vi "Convert Enum to Image.vi"(6 "picture background":picture, 8 "error in":errorcluster, 11 "Graphics":T1="info") -> (0 "error out":errorcluster, 3 "Image":picture)   [LabVIEW 2021, in "Pop-Up.lvlib" / "Popup.lvclass"]
doc: "This VI will take the input ENUM typedef for the Graphic chosen and will get its image data using the LabVIEW PNG files.\n\nInputs: +\n-Graphics [typedef combobox] - the image to look up +\n-background [2d picture] - the background color for the image\n\nOutputs: +\n-Image [2D Image] - the image data\n\n<b>Code Developed By:</b> +\nDaniel Coons +\nhttps://github.com/danielcoons/tsc-pop-up"
uses:
  Popup.lvclass
  Graphics.ctl
  Popup.lvclass/Popup.ctl
  Pop-Up.lvlib
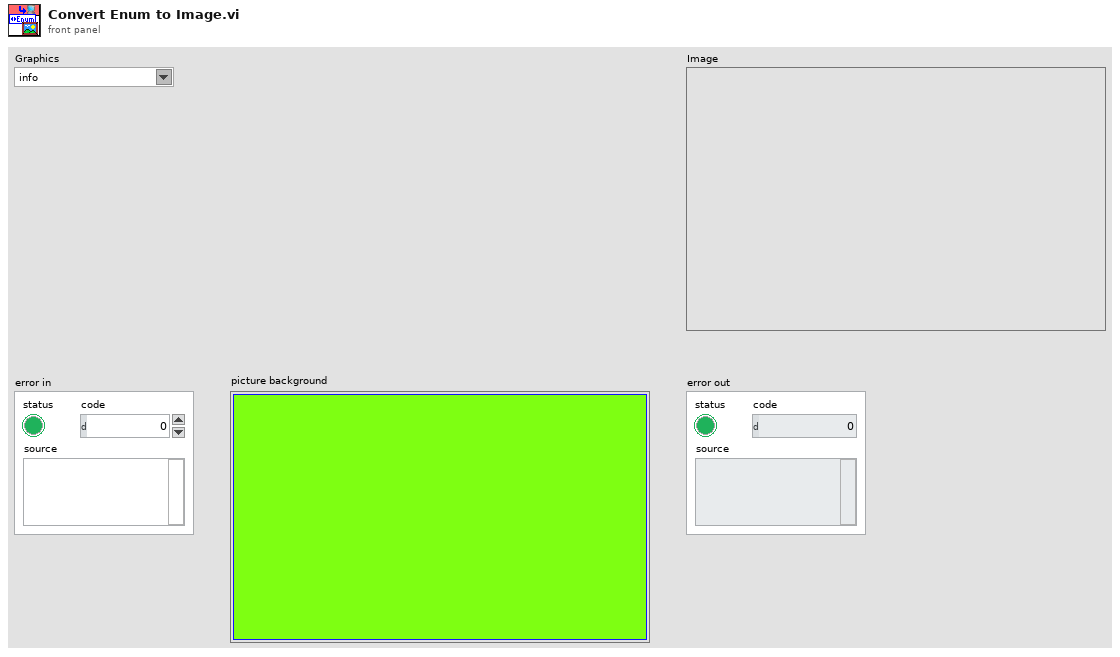
[diagram p1: front panel]
types:
  T1 = typedef "Pop-Up.lvlib/Graphics.ctl" = string
  T2 = cluster{"image type":i32, "image depth":i32, "image":u8[], "mask":u8[], "colors":u32[], "Rectangle":cluster{"left":i16, "top":i16, "right":i16, "bottom":i16}}
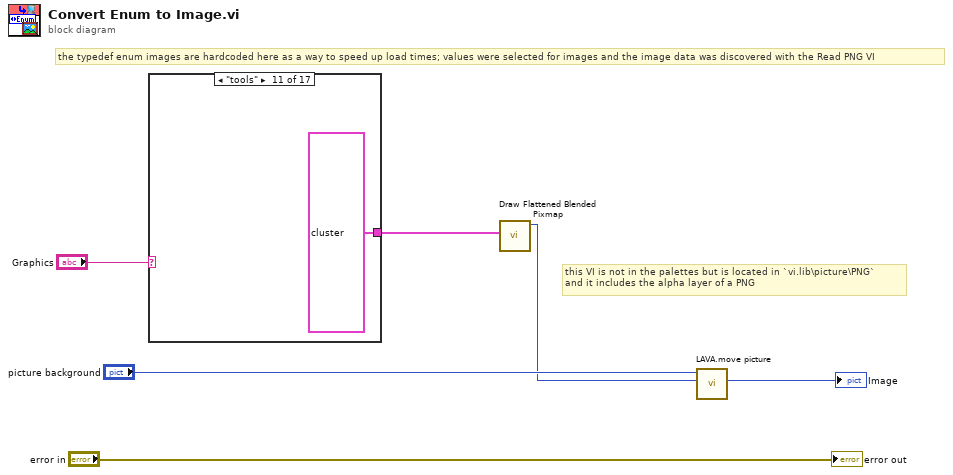
[diagram p0: block diagram]
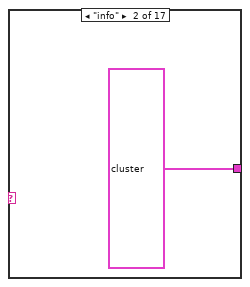
[diagram p3: hidden frame]
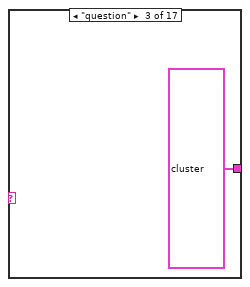
[diagram p4: hidden frame]
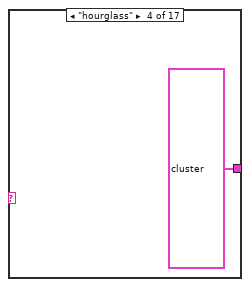
[diagram p5: hidden frame]
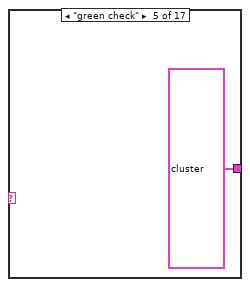
[diagram p6: hidden frame]
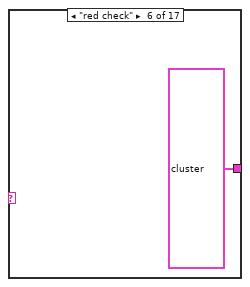
[diagram p7: hidden frame]
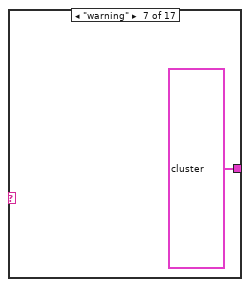
[diagram p8: hidden frame]
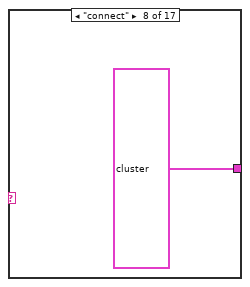
[diagram p9: hidden frame]
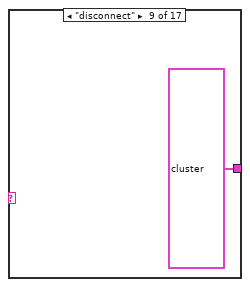
[diagram p10: hidden frame]
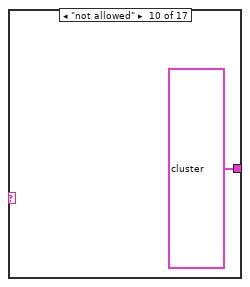
[diagram p11: hidden frame]
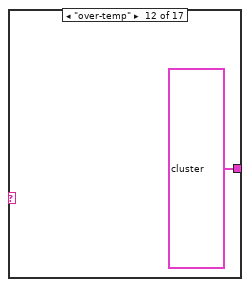
[diagram p12: hidden frame]
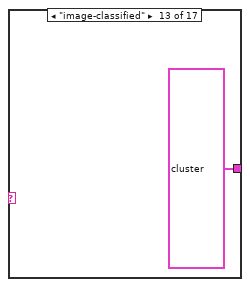
[diagram p13: hidden frame]
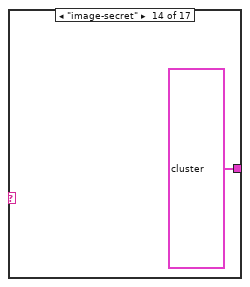
[diagram p14: hidden frame]
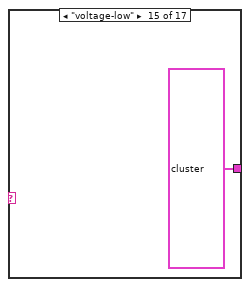
[diagram p15: hidden frame]
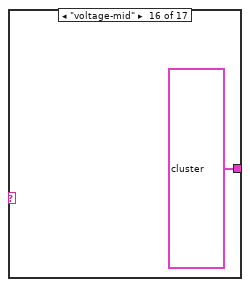
[diagram p16: hidden frame]
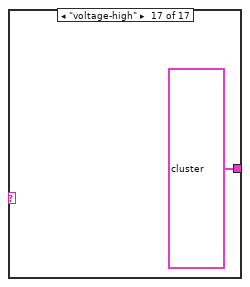
[diagram p17: hidden frame]
diagram:
  # "this VI is not in the palettes but is located in `vi.lib\\picture\\PNG`\nand it includes the alpha layer of a PNG"
  # "the typedef enum images are hardcoded here as a way to speed up load times; values were selected for images and the image data was discovered with the Read PNG VI"
  n1 = case shown="\"tools\"" "Graphics" {
    tunnel: [_ T2 {"image type"=0, "image depth"=32, "image"=array[443520 elements], "mask"=array[14256 elements], "colors"=[], "Rectangle"={"left"=0, "top"=0, "right"=420, "bottom"=264}} T2 {"image type"=0, "image depth"=32, "image"=array[443520 elements], "mask"=array[14256 elements], "colors"=[], "Rectangle"={"left"=0, "top"=0, "right"=420, "bottom"=264}} T2 {"image type"=0, "image depth"=32, "image"=array[443520 elements], "mask"=array[14256 elements], "colors"=[], "Rectangle"={"left"=0, "top"=0, "right"=420, "bottom"=264}} T2 {"image type"=0, "image depth"=32, "image"=array[443520 elements], "mask"=array[14256 elements], "colors"=[], "Rectangle"={"left"=0, "top"=0, "right"=420, "bottom"=264}} T2 {"image type"=0, "image depth"=32, "image"=array[443520 elements], "mask"=array[14256 elements], "colors"=[], "Rectangle"={"left"=0, "top"=0, "right"=420, "bottom"=264}} T2 {"image type"=0, "image depth"=32, "image"=array[443520 elements], "mask"=array[14256 elements], "colors"=[], "Rectangle"={"left"=0, "top"=0, "right"=420, "bottom"=264}} T2 {"image type"=0, "image depth"=32, "image"=array[443520 elements], "mask"=array[14256 elements], "colors"=[], "Rectangle"={"left"=0, "top"=0, "right"=420, "bottom"=264}} T2 {"image type"=0, "image depth"=32, "image"=array[443520 elements], "mask"=array[14256 elements], "colors"=[], "Rectangle"={"left"=0, "top"=0, "right"=420, "bottom"=264}} T2 {"image type"=0, "image depth"=32, "image"=array[443520 elements], "mask"=array[14256 elements], "colors"=[], "Rectangle"={"left"=0, "top"=0, "right"=420, "bottom"=264}} T2 {"image type"=0, "image depth"=32, "image"=array[443520 elements], "mask"=array[14256 elements], "colors"=[], "Rectangle"={"left"=0, "top"=0, "right"=420, "bottom"=264}} T2 {"image type"=0, "image depth"=32, "image"=array[443520 elements], "mask"=array[14256 elements], "colors"=[], "Rectangle"={"left"=0, "top"=0, "right"=420, "bottom"=264}} T2 {"image type"=0, "image depth"=32, "image"=array[443520 elements], "mask"=array[14256 elements], "colors"=[], "Rectangle"={"left"=0, "top"=0, "right"=420, "bottom"=264}} T2 {"image type"=0, "image depth"=32, "image"=array[443520 elements], "mask"=array[14256 elements], "colors"=[], "Rectangle"={"left"=0, "top"=0, "right"=420, "bottom"=264}} T2 {"image type"=0, "image depth"=32, "image"=array[443520 elements], "mask"=array[14256 elements], "colors"=[], "Rectangle"={"left"=0, "top"=0, "right"=420, "bottom"=264}} T2 {"image type"=0, "image depth"=32, "image"=array[443520 elements], "mask"=array[14256 elements], "colors"=[], "Rectangle"={"left"=0, "top"=0, "right"=420, "bottom"=264}} T2 {"image type"=0, "image depth"=32, "image"=array[443520 elements], "mask"=array[14256 elements], "colors"=[], "Rectangle"={"left"=0, "top"=0, "right"=420, "bottom"=264}}] -> w1
    frame Default {
    }
    frame "info" {
    }
    frame "question" {
    }
    frame "hourglass" {
    }
    frame "green check" {
    }
    frame "red check" {
    }
    frame "warning" {
    }
    frame "connect" {
    }
    frame "disconnect" {
    }
    frame "not allowed" {
    }
    frame "tools" {
    }
    frame "over-temp" {
    }
    frame "image-classified" {
    }
    frame "image-secret" {
    }
    frame "voltage-low" {
    }
    frame "voltage-mid" {
    }
    frame "voltage-high" {
    }
  }
  n2 = call <vilib>:"Draw Flattened Blended Pixmap.vi"("image data"=w1) -> ("new picture"=w2:picture)  [unwired: 7 in, 1 out]
  n3 = call "LAVA.move picture.vi"("Picture in"=w2, "background"="picture background") -> ("Picture out"=→"Image":picture)  [unwired: 9 in]
  "error out" <- "error in"
